vi "polymorphism example.vi"() -> ()   [LabVIEW 2018]
panel:
  out "Waveform Chart":dbl[][](graph)
  in  "Numeric":dbl
  out "Array 1 + Array 2":dbl[](array[numeric])
  out "Array 1*Scale":dbl[](array[numeric])
  out "Array 2":dbl[](array[numeric])
  out "Array 1":dbl[](array[numeric])
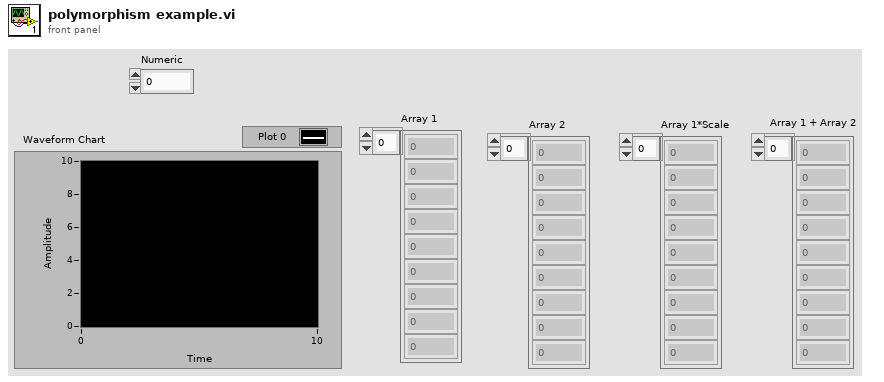
[diagram p1: front panel]
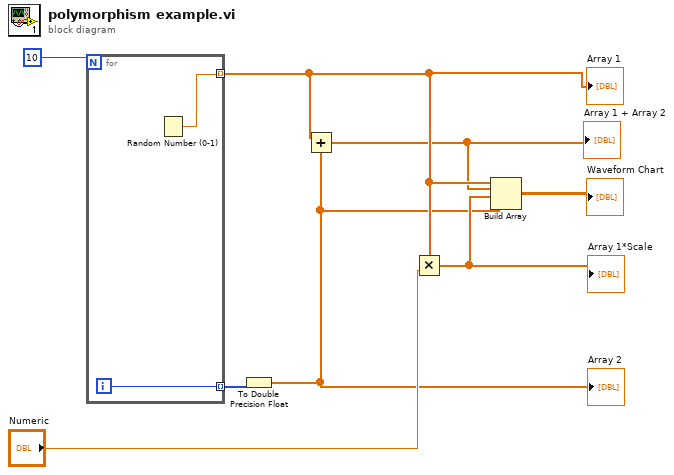
[diagram p0: block diagram]
diagram:
  n1 = for {
    N: 10 -> [_]
    tunnel: [w10] -> w6 mode=indexing
    tunnel: [w9] -> w1 mode=indexing
    i -> [w9]
    n2 = Random Number (0-1)() -> (number: 0 to 1=w10:dbl)
  }
  "Array 1" <- w6
  n3 = To Double Precision Float(number=w1) -> (double precision float=w2:dbl[])
  "Array 2" <- w2
  n4 = Add(x=w6, y=w2) -> (x+y=w4:dbl[])
  "Array 1 + Array 2" <- w4
  n5 = Multiply(x=w6, y="Numeric") -> (x*y=w5:dbl[])
  "Array 1*Scale" <- w5
  n6 = Build Array(w6, w4, w5, w2) -> (→"Waveform Chart":dbl[][])
